vi "Cleanup.vi"(8 "error in (no error)":errorcluster, 11 "App in":refnum<class "App.lvclass">) -> (0 "error out":errorcluster)   [LabVIEW 2020, in "App.lvclass"]
uses:
  App.lvclass
  App.lvclass/App.ctl
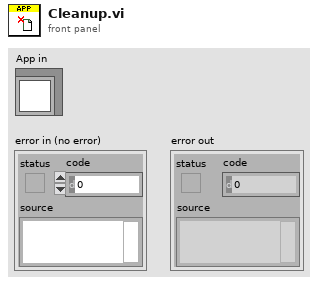
[diagram p1: front panel]
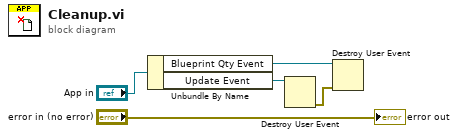
[diagram p0: block diagram]
diagram:
  n1 = Unbundle By Name("App in") -> ("Blueprint Qty Event"=w2:refnum<user-event>, "Update Event"=w3:refnum<user-event>)
  n2 = Destroy User Event(user event=w3) -> (error out=w1:errorcluster)  [unwired: 1 in]
  n3 = Destroy User Event(user event=w2, error in=w1) -> ()  [unwired: 1 out]
  "error out" <- "error in (no error)"
